vi "LimitReached.vi"(8 "error in (no error)":errorcluster, 11 "TranslationStage in":refnum<class "ArduinoTranslationStage.lvclass">) -> (0 "error out":errorcluster, 3 "TranslationStage out":refnum<class "ArduinoTranslationStage.lvclass">)   [LabVIEW 2023]
uses:
  ArduinoTranslationStage.lvclass
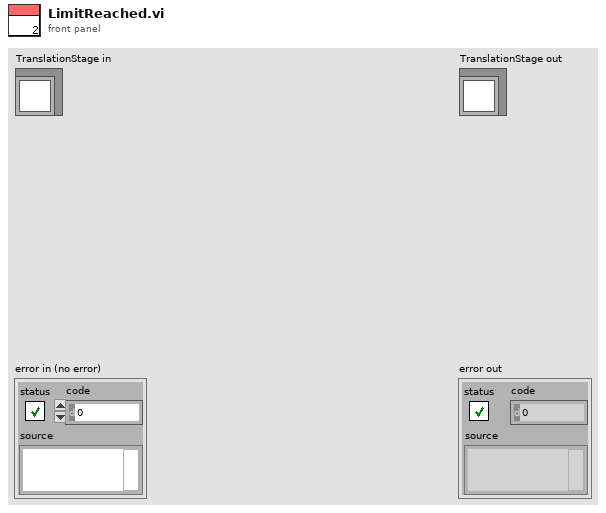
[diagram p1: front panel]
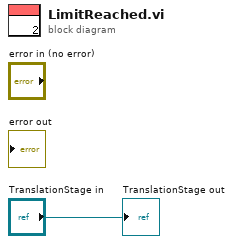
[diagram p0: block diagram]
diagram:
  "TranslationStage out" <- "TranslationStage in"
